vi "Send Message to Host.vi"(8 "error in":errorcluster, 9 "Remote UDP Listening Port":u16, 10 "Remote IP":string, 11 "UDP Message":T1) -> (0 "error out":errorcluster)   [LabVIEW 2021, in "RT Interpreter Manager.lvlib"]
doc: "_____\nCreated using DQMH Framework: Event Scripter 7.1.2.1547."
uses:
  Libraries/UDP Comms/UDP Message--cluster.ctl
  Send Message to Host Argument--cluster.ctl
  RT Interpreter Manager.lvlib
  Libraries/UDP Comms/UDP Comms.lvlib
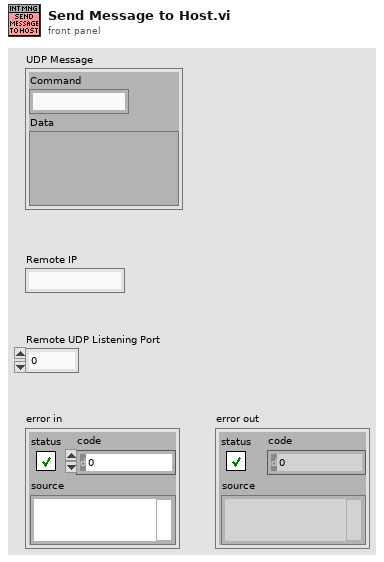
[diagram p1: front panel]
types:
  T1 = typedef "UDP Comms.lvlib/UDP Message--cluster.ctl" = cluster{"Command":string, "Data":variant}
  T2 = typedef "RT Interpreter Manager.lvlib/Send Message to Host Argument--cluster.ctl" = cluster{"UDP Message":T1, "Remote IP":string, "Remote UDP Listening Port":u16}
  T3 = typedef "RT Interpreter Manager.lvlib/Request Events--cluster.ctl" = cluster{"Stop Module":refnum<user-event>, "Show Panel":refnum<user-event>, "Hide Panel":refnum<user-event>, "Get Module Execution Status":refnum<user-event>, "Show Diagram":refnum<user-event>, "Private.Get Config":refnum<user-event>, "Private.Open UDP":refnum<user-event>, "Private.Start Read Messages from Host HL":refnum<user-event>, "Private.New Host Connection":refnum<user-event>, "Private.Send Message to Host":refnum<user-event>, "Private.Delete Host Connection":refnum<user-event>}
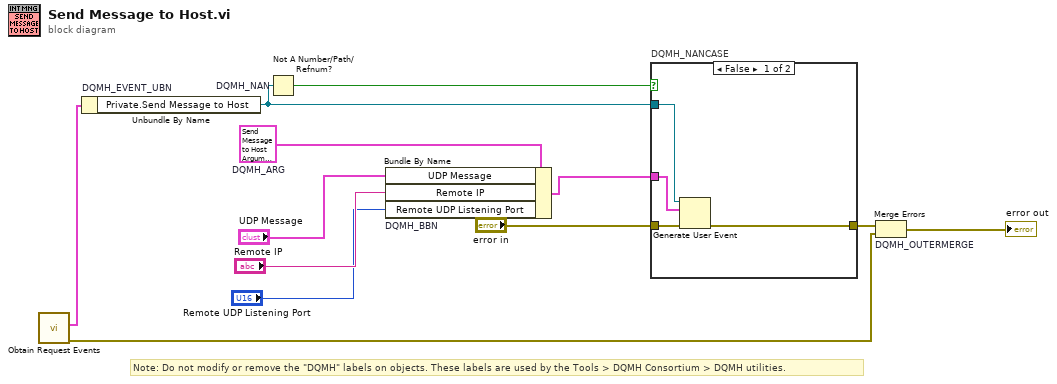
[diagram p0: block diagram]
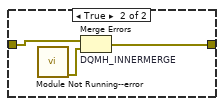
[diagram p2: hidden frame]
diagram:
  w6 = T2 {"UDP Message"={"Command"="", "Data"=variant}, "Remote IP"="", "Remote UDP Listening Port"=0}  # DQMH_ARG
  # "Note: Do not modify or remove the \"DQMH\" labels on objects. These labels are used by the Tools > DQMH Consortium > DQMH utilities."
  n1 = call "Obtain Request Events.vi"() -> ("error out"=w4:errorcluster, "RT Interpreter Manager Request Events"=w3:T3)  [unwired: 10 in]
  n2 = Unbundle By Name "DQMH_EVENT_UBN"(w3) -> ("Private.Send Message to Host"=w8:refnum<user-event>)
  n3 = Not A Number/Path/Refnum? "DQMH_NAN"(number/path/refnum=w8) -> (NaN/Path/Refnum?=w9:bool)
  n4 = Bundle By Name "DQMH_BBN"(cluster=w6, "UDP Message"="UDP Message", "Remote IP"="Remote IP", "Remote UDP Listening Port"="Remote UDP Listening Port") -> (w10:T2)
  n5 = case "DQMH_NANCASE" shown="False" w9 {
    tunnel: "error in" -> [w16 w19]
    tunnel: [w15 w18] -> w7
    tunnel: w8 -> [w14 _]
    tunnel: w10 -> [w13 _]
    frame False {
      n6 = Generate User Event(user event=w14, event data cluster=w13, error in=w16) -> (error out=w15:errorcluster)  [unwired: 1 in, 1 out]
    }
    frame True {
      n7 = call "Module Not Running--error.vi"() -> ("error out"=w17:errorcluster)  [unwired: 11 in]
      n8 = Merge Errors "DQMH_INNERMERGE"(w19, w17) -> (w18:errorcluster)
    }
  }
  n9 = Merge Errors "DQMH_OUTERMERGE"(w7, w4) -> (→"error out":errorcluster)
